vi "Path_2_String.vi"(1 "Real Path":path) -> (0 "Path String":string)   [LabVIEW 2015]
uses:
  Globals/Constants_global.vi
  Globals/Preference_global.vi
panel:
  in  "POSIXFormattedPseudopath (F)":bool
  out "Data Folder":path
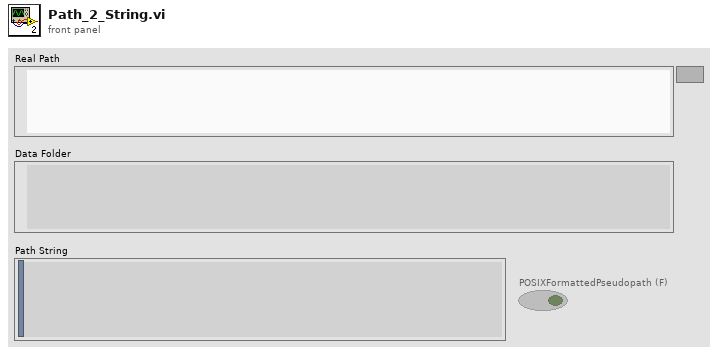
[diagram p1: front panel]
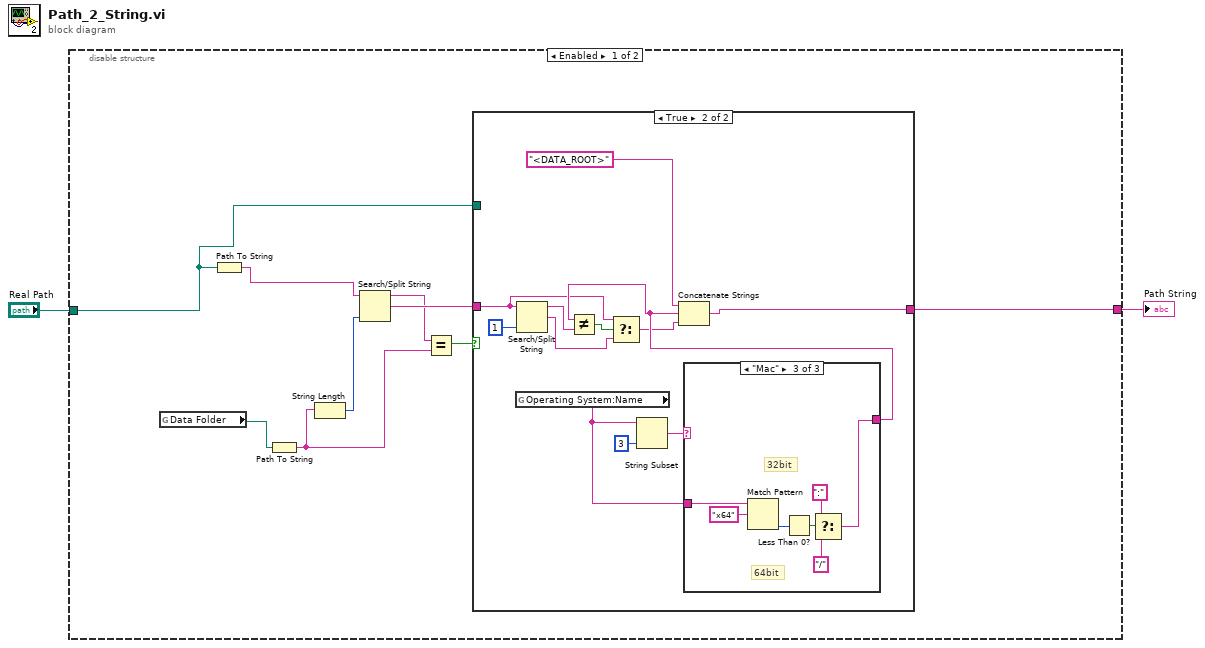
[diagram p0: block diagram]
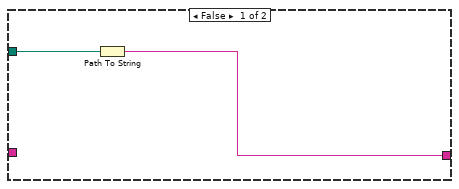
[diagram p2: hidden frame]
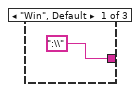
[diagram p3: hidden frame]
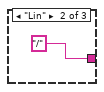
[diagram p4: hidden frame]
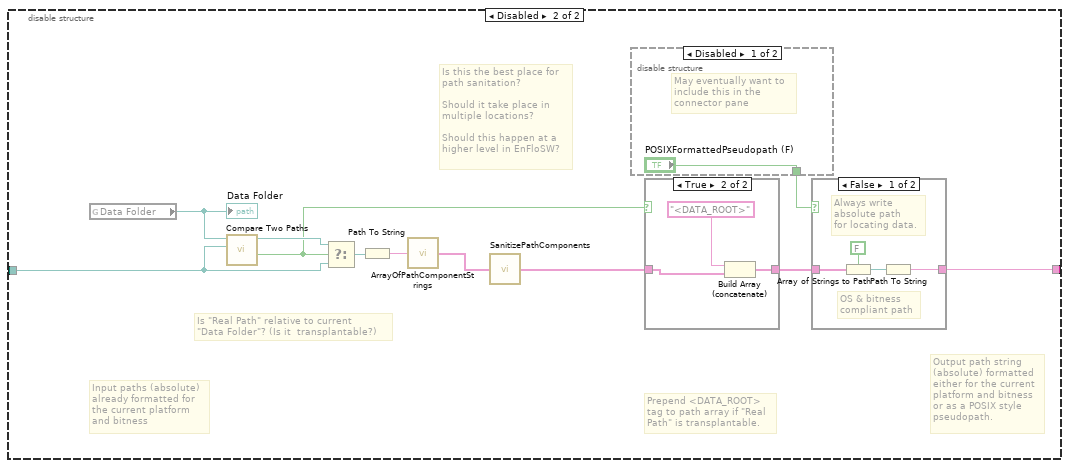
[diagram p5: hidden frame]
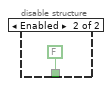
[diagram p6: hidden frame]
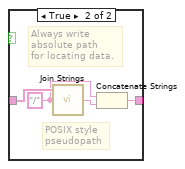
[diagram p7: hidden frame]
diagram:
  n1 = disable-structure shown="Enabled" {
    disable-tunnel: "Real Path" -> [w4 w36]
    disable-tunnel: [w3 w35] -> w1
    frame Enabled {
      n2 = global read "Constants_global.vi" "Data Folder"() -> (w5:path)
      n3 = Path To String(path=w4) -> (string=w7:string)
      n4 = Path To String(path=w5) -> (string=w8:string)
      n5 = String Length(string=w8) -> (length=w6:i32)
      n6 = Search/Split String(string=w7, offset (0)=w6) -> (substring before match=w10:string, match + rest of string=w11:string)  [unwired: 1 in, 1 out]
      n7 = Equal?(x=w10, y=w8) -> (x = y?=w9:bool)
      n8 = case shown="True" w9 {
        tunnel: w4 -> [w13 _]
        tunnel: [w12 w24] -> w3
        tunnel: w11 -> [_ w15]
        frame False {
          n9 = Path To String(path=w13) -> (string=w12:string)
        }
        frame True {
          n10 = global read "Preference_global.vi" "Operating System:Name"() -> (w14:string)
          n11 = Search/Split String(string=w15, offset (0)=1 ("length (rest)")) -> (substring before match=w17:string, match + rest of string=w18:string)  [unwired: 2 out]
          n12 = String Subset(string=w14, length (rest)=3 ("length (rest)")) -> (substring=w22:string)  [unwired: 1 out]
          n13 = case shown="\"Mac\"" w22 {
            tunnel: [":\\" "/" w29] -> w20
            tunnel: w14 -> [_ _ w34]
            frame "Win", Default {
            }
            frame "Lin" {
            }
            frame "Mac" {
              # "64bit"
              # "32bit"
              n14 = Match Pattern(string=w34, regular expression="x64") -> (offset past match=w32:i32)  [unwired: 1 in, 3 out]
              n15 = Less Than 0?(x=w32) -> (x < 0?=w31:bool)
              n16 = Select(t=":", s=w31, f="/") -> (s? t:f=w29:string)
            }
          }
          n17 = Not Equal?(x=w20, y=w17) -> (x != y?=w19:bool)
          n18 = Select(t=w15, s=w19, f=w18) -> (s? t:f=w16:string)
          n19 = Concatenate Strings("<DATA_ROOT>", w20, w16) -> (w24:string)
        }
      }
    }
    frame Disabled {
      # "Output path string\n(absolute) formatted\neither for the current\nplatform and bitness\nor as a POSIX style\npseudopath."
      # "Is this the best place for\npath sanitation?\n\nShould it take place in\nmultiple locations?\n\nShould this happen at a\nhigher level in EnFloSW?"
      # "Input paths (absolute)\nalready formatted for\nthe current platform \nand bitness"
      # "Is \"Real Path\" relative to current\n\"Data Folder\"? (Is it  transplantable?)"
      # "Prepend <DATA_ROOT>\ntag to path array if \"Real\nPath\" is transplantable."
      # "Input paths (absolute)\nalready formatted for\nthe current platform \nand bitness"
      n20 = global read "Constants_global.vi" "Data Folder"() -> (w37:path)
      "Data Folder" <- w37
      n21 = call <vilib>:"Compare Two Paths.vi"("Path 2"=w36, "Path 1"=w37) -> ("Path 2 Relative to Path 1?"=w38:bool, "Relative Path from 1 to 2"=w39:path)  [unwired: 6 in, 2 out]
      n22 = Select(t=w39, s=w38, f=w36) -> (s? t:f=w40:path)
      n23 = Path To String(path=w40) -> (string=w43:string)
      n24 = call "ArrayOfPathComponentStrings.vi"("PathStringIn"=w43) -> ("ArrayOfPathComponentStringsOut"=w45:string[])
      n25 = call "SanitizePathComponents.vi"("PathComponentsIn"=w45) -> ("SanitizedComponentsOut"=w44:string[])
      n26 = disable-structure shown="Disabled" {
        disable-tunnel: ["POSIXFormattedPseudopath (F)" FALSE ("POSIXFormattedPseudopath (F)")] -> w42
        frame Disabled {
          # "May eventually want to\ninclude this in the\nconnector pane"
        }
        frame Enabled {
        }
      }
      n27 = case shown="True" w38 {
        tunnel: [w56 w58] -> w41
        tunnel: w44 -> [w56 w57]
        frame False {
        }
        frame True {
          n28 = Build Array (concatenate)("<DATA_ROOT>", w57) -> (w58:string[])
        }
      }
      n29 = case shown="False" w42 {
        tunnel: w41 -> [w48 w55]
        tunnel: [w49 w54] -> w35
        frame False {
          # "OS & bitness\ncompliant path"
          # "Always write\nabsolute path\nfor locating data."
          n30 = Array of Strings to Path(0:w48, 1:FALSE ("relative")) -> (2:w50:path)
          n31 = Path To String(path=w50) -> (string=w49:string)
        }
        frame True {
          w52 = "/" ("Separator (,)")
          # "POSIX style\npseudopath"
          # "Always write\nabsolute path\nfor locating data."
          n32 = call <vilib>:"Join Strings.vi"("Separator (,)"=w52, "Strings In"=w55) -> ("String"=w53:string)  [unwired: 1 in]
          n33 = Concatenate Strings(w52, w53) -> (w54:string)
        }
      }
    }
  }
  "Path String" <- w1
